vi "Get FPGA Bitfile.vi"(8 "error in":errorcluster, 10 "Target.Type":T1, 11 "VS Engine Interface in":refnum<class "VS Engine Interface.lvclass">) -> (0 "error out":errorcluster, 2 "Path":path, 3 "VS Engine Interface out":refnum<class "VS Engine Interface.lvclass">)   [LabVIEW 2024, in "VS Engine Abstraction.lvlib" / "VS Engine Interface.lvclass"]
uses:
  VS Engine Interface.lvclass
  <vilib>/NI VeriStand/Custom Device API/Custom Device Target Type.ctl
  <vilib>/NI VeriStand/Custom Device API/Custom Device API.lvlib
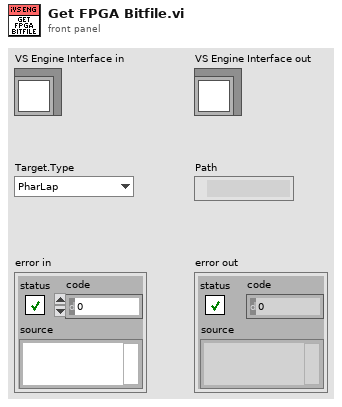
[diagram p1: front panel]
types:
  T1 = typedef "Custom Device API.lvlib/Custom Device Target Type.ctl" = enum16{"PharLap", "VxWorks", "Windows", "Linux_32_ARM", "Linux_x64"}
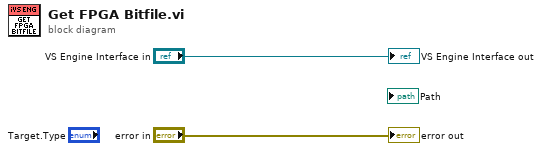
[diagram p0: block diagram]
diagram:
  "error out" <- "error in"
  "VS Engine Interface out" <- "VS Engine Interface in"
